vi "Write Keep Original.vi"(8 "error in (no error)":errorcluster, 10 "Keep Original":bool, 11 "Remap Bus in":refnum<class "Remap Bus.lvclass">) -> (0 "error out":errorcluster, 3 "Remap Bus out":refnum<class "Remap Bus.lvclass">)   [LabVIEW 2021, in "Remap Bus.lvclass"]
uses:
  Remap Bus.lvclass
  Remap Bus.lvclass/Remap Bus.ctl
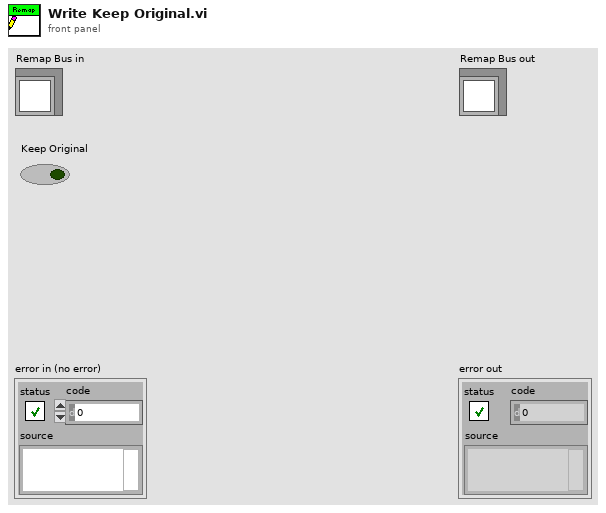
[diagram p1: front panel]
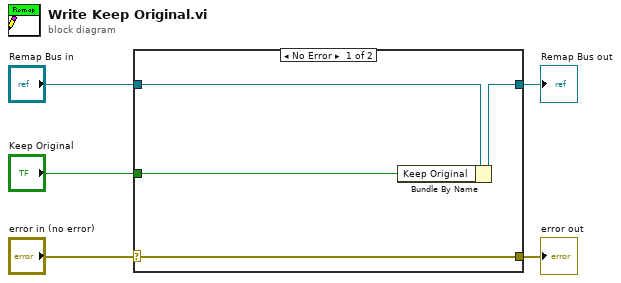
[diagram p0: block diagram]
diagram:
  n1 = case shown="No Error" "error in (no error)" {
    selector: "error in (no error)" -> [w9 w10]
    tunnel: [w9 w10] -> w4
    tunnel: [w7 w11] -> w2
    tunnel: "Remap Bus in" -> [w8 w11]
    tunnel: "Keep Original" -> [w6 _]
    frame No Error {
      n2 = Bundle By Name(cluster=w8, "Keep Original"=w6) -> (w7:refnum<class "Remap Bus.lvclass">)
    }
    frame Error {
    }
  }
  "error out" <- w4
  "Remap Bus out" <- w2
